vi "病人基本信息编辑 (早癌）.vi"() -> ()   [LabVIEW 2018]
uses:
  <vilib>/Utility/NIReport.llb/Report Type.ctl
  <vilib>/Utility/NIReport.llb/Append Report Text (str wrap).vi
  <vilib>/Utility/NIReport.llb/NI_report.lvclass
  <vilib>/Utility/NIReport.llb/NI_ReportGenerationCore.lvlib
panel:
  in  "报表模板名称":string caption="报表模板名称（必须在“\\报表模板”目录下）"
  in  "主页按钮":bool
  in  "初步检查所见：":string
  in  "打开按钮":bool
  in  "保存按钮":bool
  in  "来源：":string
  in  "床号：":string
  in  "科别：":string
  in  "年龄：":string
  in  "性别：":string
  in  "姓名：":string
  in  "检查号：":string
  in  "病历号：":string
  in  "住院号：":string
  in  "门诊号：":string
  # "病人基本信息"
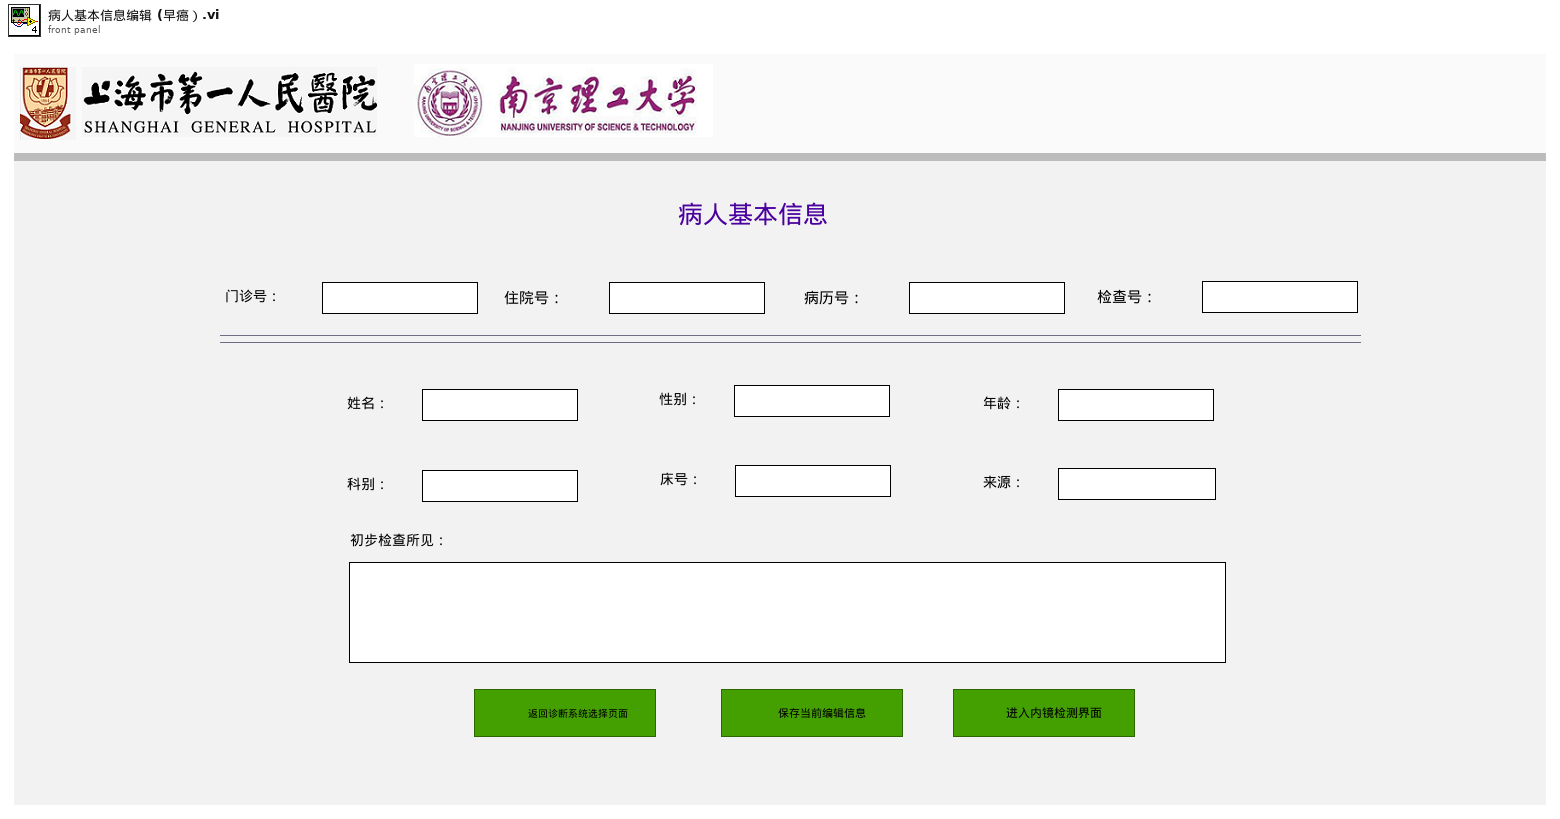
[diagram p1: front panel]
types:
  T1 = enum16{"maximized", "minimized", "normal", "no change"}
  T2 = cluster{"position (Excel)":cluster{"row":i32, "column":i32}, "name (Excel)":string, "bookmark (Word)":string}
  T3 = typedef "NI_ReportGenerationCore.lvlib/Report Type.ctl" = enum16{"HTML", "Word", "Excel"}
  T4 = enum32{"Invalid", "Standard", "Closed", "Hidden", "Minimized", "Maximized"}
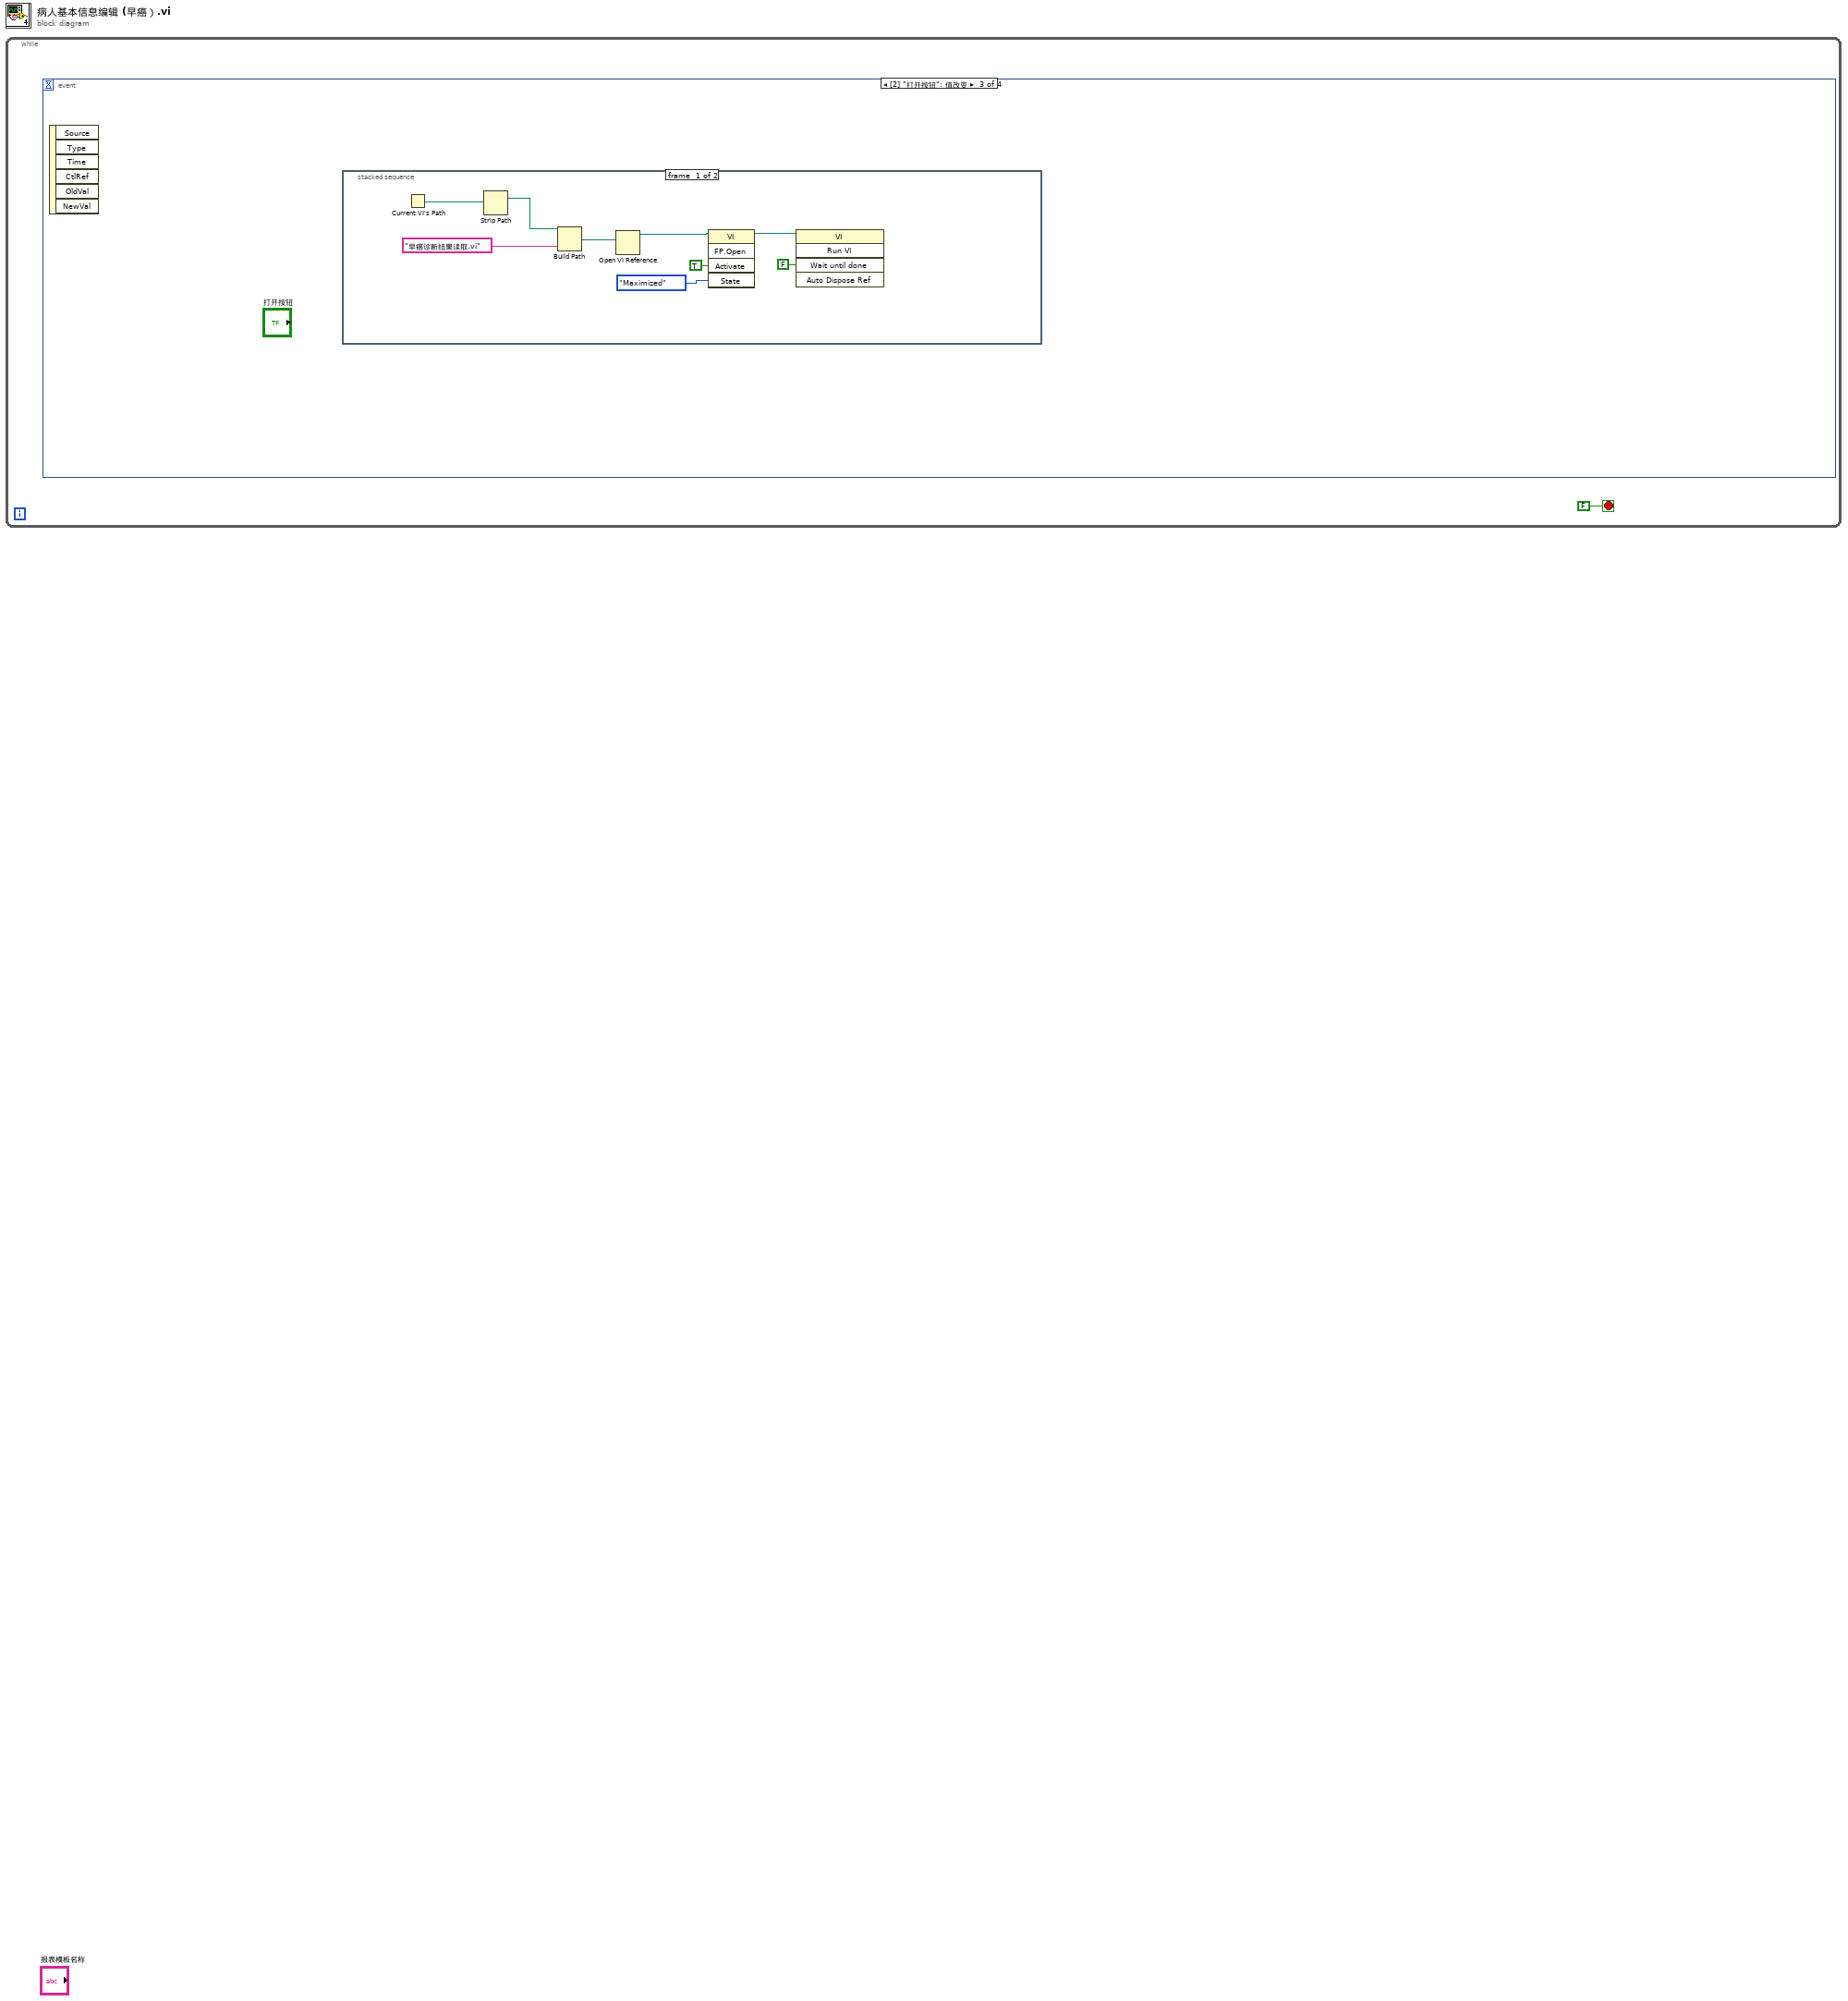
[diagram p0: block diagram]
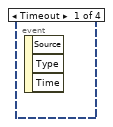
[diagram p2: hidden frame]
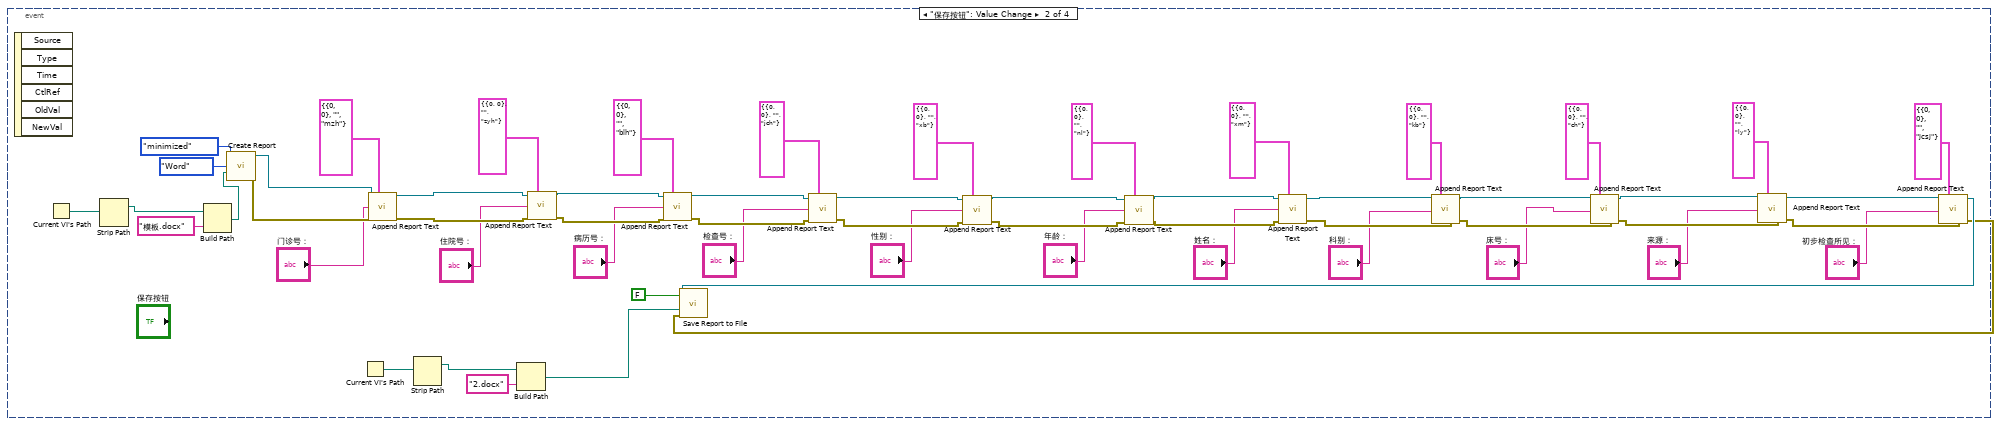
[diagram p3: hidden frame]
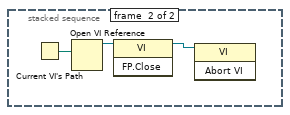
[diagram p4: hidden frame]
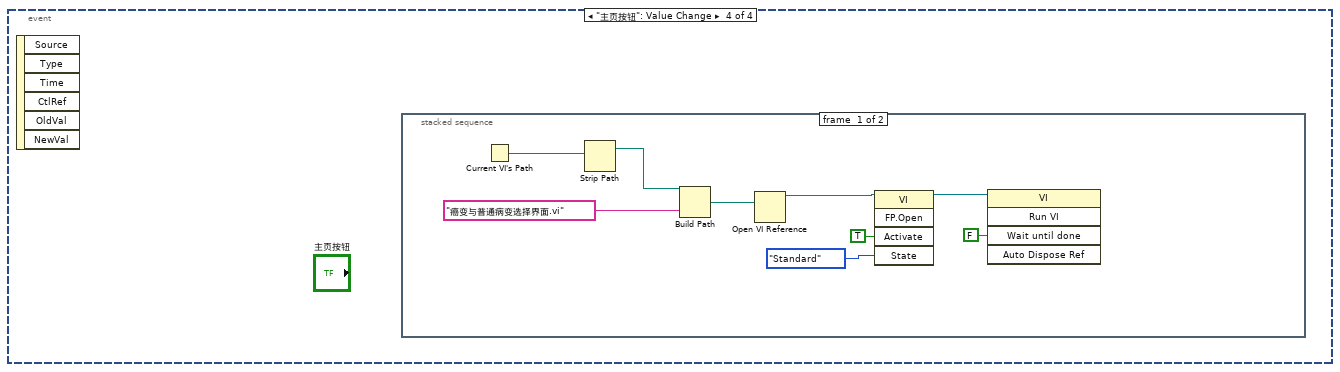
[diagram p5: hidden frame]
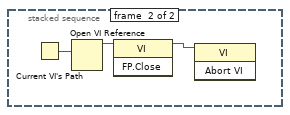
[diagram p6: hidden frame]
diagram:
  n1 = while {
    stop <- FALSE stop-if-true
    n2 = event shown="[2] \"打开按钮\": 值改变" {
      selector: _ -> [_ _ _ _]
      dyn-events: _ -> [_ _ _ _]
      timeout: _ -> [_ _ _ _]
      event Timeout {
        n3 = event-data() -> ()  [unwired: 1 in, 3 out]
      }
      event "保存按钮": Value Change {
        n4 = event-data() -> ()  [unwired: 1 in, 6 out]
        n5 = Current VI's Path() -> (path=w55:path)
        n6 = Strip Path(path=w55) -> (stripped path=w54:path)  [unwired: 1 out]
        n7 = Build Path(base path=w54, name or relative path="模板.docx" ("名称或相对路径")) -> (appended path=w58:path)
        n8 = call <vilib>:"Create Report.vi"("window state (normal)"=T1."minimized", "report type"=Report_Type."Word" ("Report Type"), "template (empty)"=w58) -> ("report out"=w57:refnum<class "NI_report.lvclass">, "error out"=w56:errorcluster)  [unwired: 11 in]
        n9 = Current VI's Path() -> (path=w53:path)
        n10 = call-poly <vilib>:"Append Report Text.vi"("report in"=w57, "MS Office parameters"=T2 {"position (Excel)"={"row"=0, "column"=0}, "name (Excel)"="", "bookmark (Word)"="mzh"}, "text"="门诊号：", "error in (no error)"=w56) -> ("report out"=w49:refnum<class "NI_report.lvclass">, "error out"=w50:errorcluster)  [unwired: 8 in, 2 out]
        n11 = Strip Path(path=w53) -> (stripped path=w52:path)  [unwired: 1 out]
        n12 = Build Path(base path=w52, name or relative path="2.docx" ("名称或相对路径")) -> (appended path=w51:path)
        n13 = call-poly <vilib>:"Append Report Text.vi"("report in"=w49, "MS Office parameters"=T2 {"position (Excel)"={"row"=0, "column"=0}, "name (Excel)"="", "bookmark (Word)"="zyh"}, "text"="住院号：", "error in (no error)"=w50) -> ("report out"=w41:refnum<class "NI_report.lvclass">, "error out"=w40:errorcluster)  [unwired: 8 in, 2 out]
        n14 = call-poly <vilib>:"Append Report Text.vi"("report in"=w41, "MS Office parameters"=T2 {"position (Excel)"={"row"=0, "column"=0}, "name (Excel)"="", "bookmark (Word)"="blh"}, "text"="病历号：", "error in (no error)"=w40) -> ("report out"=w38:refnum<class "NI_report.lvclass">, "error out"=w37:errorcluster)  [unwired: 8 in, 2 out]
        n15 = call-poly <vilib>:"Append Report Text.vi"("report in"=w38, "MS Office parameters"=T2 {"position (Excel)"={"row"=0, "column"=0}, "name (Excel)"="", "bookmark (Word)"="jch"}, "text"="检查号：", "error in (no error)"=w37) -> ("report out"=w35:refnum<class "NI_report.lvclass">, "error out"=w34:errorcluster)  [unwired: 8 in, 2 out]
        n16 = call-poly <vilib>:"Append Report Text.vi"("report in"=w35, "MS Office parameters"=T2 {"position (Excel)"={"row"=0, "column"=0}, "name (Excel)"="", "bookmark (Word)"="xb"}, "text"="性别：", "error in (no error)"=w34) -> ("report out"=w32:refnum<class "NI_report.lvclass">, "error out"=w31:errorcluster)  [unwired: 8 in, 2 out]
        n17 = call-poly <vilib>:"Append Report Text.vi"("report in"=w32, "MS Office parameters"=T2 {"position (Excel)"={"row"=0, "column"=0}, "name (Excel)"="", "bookmark (Word)"="nl"}, "text"="年龄：", "error in (no error)"=w31) -> ("report out"=w29:refnum<class "NI_report.lvclass">, "error out"=w28:errorcluster)  [unwired: 8 in, 2 out]
        n18 = call-poly <vilib>:"Append Report Text.vi"("report in"=w29, "MS Office parameters"=T2 {"position (Excel)"={"row"=0, "column"=0}, "name (Excel)"="", "bookmark (Word)"="xm"}, "text"="姓名：", "error in (no error)"=w28) -> ("report out"=w26:refnum<class "NI_report.lvclass">, "error out"=w25:errorcluster)  [unwired: 8 in, 2 out]
        n19 = call-poly <vilib>:"Append Report Text.vi"("report in"=w26, "MS Office parameters"=T2 {"position (Excel)"={"row"=0, "column"=0}, "name (Excel)"="", "bookmark (Word)"="kb"}, "text"="科别：", "error in (no error)"=w25) -> ("report out"=w23:refnum<class "NI_report.lvclass">, "error out"=w22:errorcluster)  [unwired: 8 in, 2 out]
        n20 = call-poly <vilib>:"Append Report Text.vi"("report in"=w23, "MS Office parameters"=T2 {"position (Excel)"={"row"=0, "column"=0}, "name (Excel)"="", "bookmark (Word)"="ch"}, "text"="床号：", "error in (no error)"=w22) -> ("report out"=w20:refnum<class "NI_report.lvclass">, "error out"=w19:errorcluster)  [unwired: 8 in, 2 out]
        n21 = call-poly <vilib>:"Append Report Text.vi"("report in"=w20, "MS Office parameters"=T2 {"position (Excel)"={"row"=0, "column"=0}, "name (Excel)"="", "bookmark (Word)"="ly"}, "text"="来源：", "error in (no error)"=w19) -> ("report out"=w7:refnum<class "NI_report.lvclass">, "error out"=w6:errorcluster)  [unwired: 8 in, 2 out]
        n22 = call-poly <vilib>:"Append Report Text.vi"("report in"=w7, "MS Office parameters"=T2 {"position (Excel)"={"row"=0, "column"=0}, "name (Excel)"="", "bookmark (Word)"="jcsj"}, "text"="初步检查所见：", "error in (no error)"=w6) -> ("report out"=w4:refnum<class "NI_report.lvclass">, "error out"=w3:errorcluster)  [unwired: 8 in, 2 out]
        n23 = call-dynamic "Save Report to File.vi"("report in"=w4, "report file path"=w51, "prompt to replace? (F)"=FALSE, "error in (no error)"=w3) -> ()  [unwired: 10 in, 2 out]
      }
      event "打开按钮": Value Change {
        n24 = event-data() -> ()  [unwired: 1 in, 6 out]
        n25 = stacked-sequence {
          frame #0 {
            n26 = Current VI's Path() -> (path=w65:path)
            n27 = Strip Path(path=w65) -> (stripped path=w66:path)  [unwired: 1 out]
            n28 = Build Path(base path=w66, name or relative path="早癌诊断结果读取.vi" ("名称或相对路径")) -> (appended path=w67:path)
            n29 = Open VI Reference(vi path=w67) -> (vi reference=w63:refnum<vi>)  [unwired: 5 in, 1 out]
            n30 = invoke class="VI" method="FP.Open"(reference=w63, "Activate"=TRUE ("激活？"), "State"=T4."Maximized" ("状态")) -> (reference out=w64:refnum<vi>)  [unwired: 2 in, 4 out]
            n31 = invoke class="VI" method="Run VI"(reference=w64, "Wait until done"=FALSE ("结束前等待")) -> ()  [unwired: 3 in, 5 out]
          }
          frame #1 {
            n32 = Current VI's Path() -> (path=w70:path)
            n33 = Open VI Reference(vi path=w70) -> (vi reference=w69:refnum<vi>)  [unwired: 5 in, 1 out]
            n34 = invoke class="VI" method="FP.Close"(reference=w69) -> (reference out=w68:refnum<vi>)  [unwired: 2 in, 2 out]
            n35 = invoke class="VI" method="Abort VI"(reference=w68) -> ()  [unwired: 2 in, 3 out]
          }
        }
      }
      event "主页按钮": Value Change {
        n36 = event-data() -> ()  [unwired: 1 in, 6 out]
        n37 = stacked-sequence {
          frame #0 {
            n38 = Current VI's Path() -> (path=w77:path)
            n39 = Strip Path(path=w77) -> (stripped path=w78:path)  [unwired: 1 out]
            n40 = Build Path(base path=w78, name or relative path="癌变与普通病变选择界面.vi" ("名称或相对路径")) -> (appended path=w79:path)
            n41 = Open VI Reference(vi path=w79) -> (vi reference=w75:refnum<vi>)  [unwired: 5 in, 1 out]
            n42 = invoke class="VI" method="FP.Open"(reference=w75, "Activate"=TRUE ("激活？"), "State"=T4."Standard" ("状态")) -> (reference out=w76:refnum<vi>)  [unwired: 2 in, 4 out]
            n43 = invoke class="VI" method="Run VI"(reference=w76, "Wait until done"=FALSE ("结束前等待")) -> ()  [unwired: 3 in, 5 out]
          }
          frame #1 {
            n44 = Current VI's Path() -> (path=w82:path)
            n45 = Open VI Reference(vi path=w82) -> (vi reference=w81:refnum<vi>)  [unwired: 5 in, 1 out]
            n46 = invoke class="VI" method="FP.Close"(reference=w81) -> (reference out=w80:refnum<vi>)  [unwired: 2 in, 2 out]
            n47 = invoke class="VI" method="Abort VI"(reference=w80) -> ()  [unwired: 2 in, 3 out]
          }
        }
      }
    }
  }
